vi "WindowLockMonitor.vi"() -> ()   [LabVIEW 2017]
uses:
  <vilib>/Platform/TimedLoop/XDataNode/timing_clust.ctl
  <vilib>/Platform/TimedLoop/XDataNode/nitl_modes.ctl
  <vilib>/Platform/TimedLoop/XDataNode/wakeup.ctl
  <vilib>/DAQmx/read.llb/DAQmx Read (Analog 1D DBL NChan 1Samp).vi
  <vilib>/DAQmx/create/channels.llb/DAQmx Create Channel (AI-Current-Basic).vi
  <vilib>/DAQmx/create/channels.llb/DAQmx Create Channel (AI-Voltage-Basic).vi
  <vilib>/DAQmx/miscellaneous.llb/DAQmx Fill In Error Info.vi
  <vilib>/platform/TimedLoop/XDataNode/XDataNode.xnode
  <vilib>/Platform/TimedLoop/XDataNode/XDNodeRunTimeDep.lvlib
panel:
  out "Distance":dbl format="%#_6f"
  out "Volte L2":dbl(graph)
  out "Volte L1":dbl(graph)
  out "Distance":dbl(graph)
  out "Force":dbl(graph)
  out "error out 2":errorcluster
  in  "stop":bool
  out "error out":errorcluster
  # "A."
  # "A."
  # "mm."
  # "V"
  # "V"
  # "WINDOW LOCK/UNLOCK"
  # "WINDOW LOCK/UNLOCK"
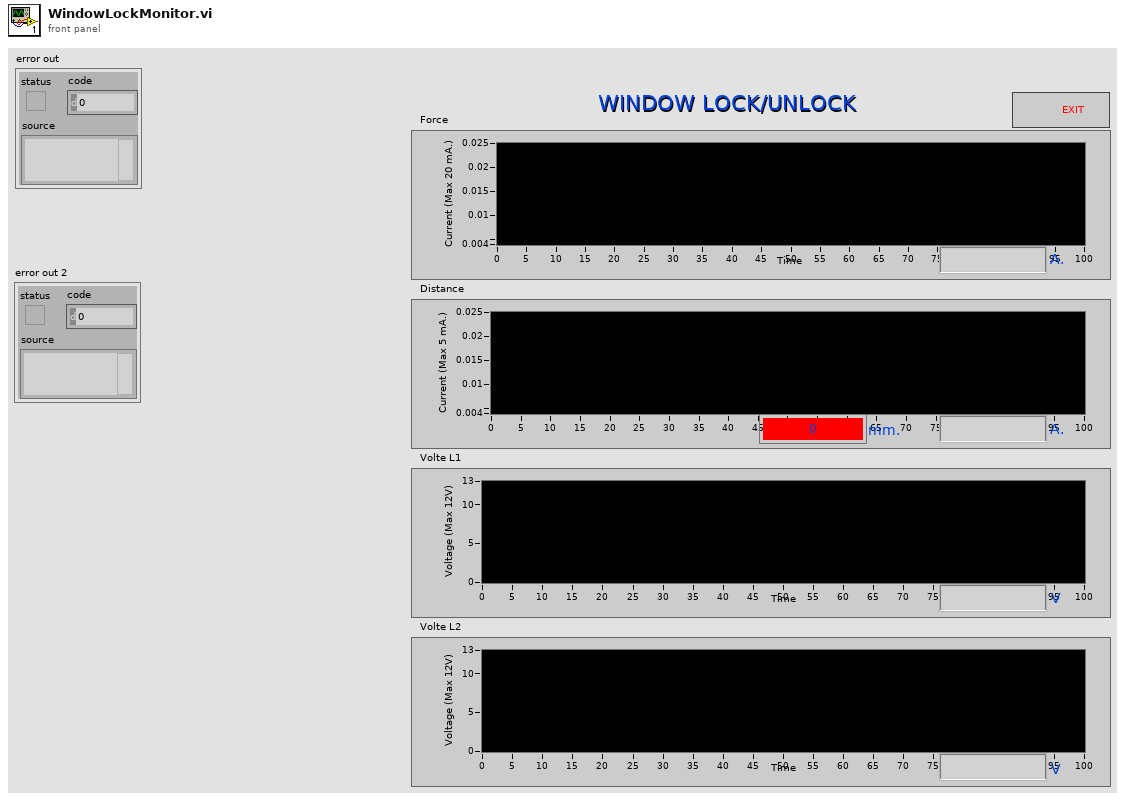
[diagram p1: front panel]
types:
  T1 = typedef "XDNodeRunTimeDep.lvlib/timing_clust.ctl" = cluster{"Expected End [f-1]":u64, "Actual End [f-1]":u64, "Finished Late? [f-1]":bool, "Expected End [i-1]":u64, "Actual End [i-1]":u64, "Finished Late? [i-1]":bool, "Expected Start [i]":u64, "Actual Start [i]":u64, "Expected Start [f]":u64, "Actual Start [f]":u64, "Source Name":string, "Structure Name":string, "Period":i64, "Deadline":i64, "Offset":i64, "Start":i64, "Priority":i32, "Timeout":i32, "Mode":T2, "Wakeup Reason":T3, "Error":errorcluster, "Source Type":string, "Secondary Source Type":string, "Global End Time":u64, "Global Start Time":u64, "Frame Duration":u64, "Iteration Duration":u64, "Assigned CPU":i32, "I/O Scan Engine Mode":u32}
  T2 = typedef "XDNodeRunTimeDep.lvlib/nitl_modes.ctl" = enum32{"No Change", "Process missed periods, maintain original phase", "Discard missed periods, maintain original phase", "Process missed periods, ignore original phase", "Discard missed periods, ignore original phase"}
  T3 = typedef "XDNodeRunTimeDep.lvlib/wakeup.ctl" = enum32{"Normal", "Aborted", "Asynchronous wakeup", "Timing source error", "Timed loop error", "Timeout"}
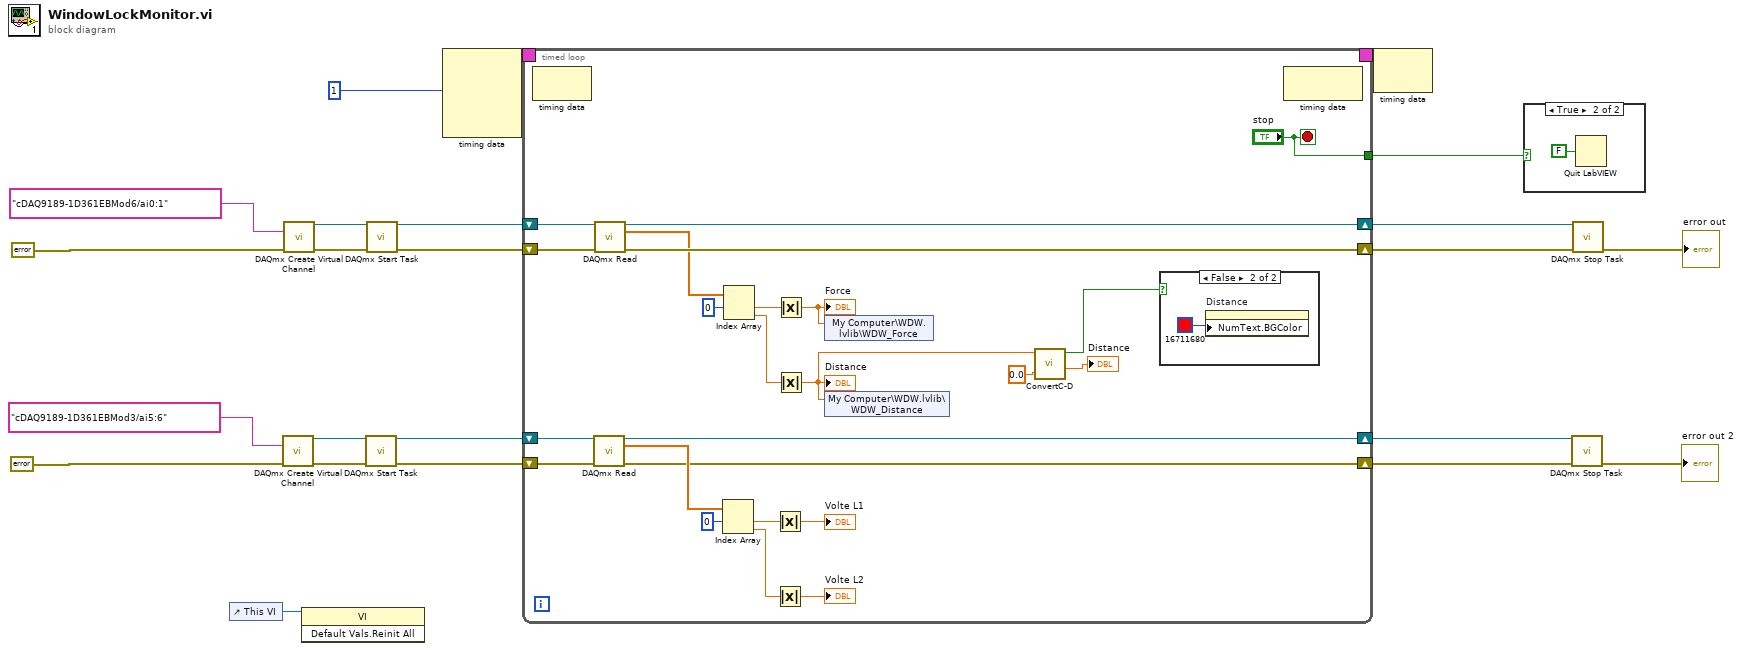
[diagram p0: block diagram]
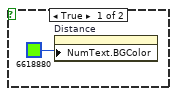
[diagram p3: hidden frame]
diagram:
  n1 = control-ref of="This VI"() -> (w11:refnum<vi>)
  n2 = call-poly <vilib>:"DAQmx Create Virtual Channel.vi"("physical channels"=tag "cDAQ9189-1D361EBMod3/ai5:6", "error in"=errorcluster {"status"=FALSE, "code"=0, "source"=""} ("error constant")) -> ("task out"=w6:refnum<k21>, "error out"=w7:errorcluster)  [unwired: 12 in]
  n3 = call-poly <vilib>:"DAQmx Create Virtual Channel.vi"("physical channels"=tag "cDAQ9189-1D361EBMod6/ai0:1", "error in"=errorcluster {"status"=FALSE, "code"=0, "source"=""} ("error constant")) -> ("task out"=w22:refnum<k21>, "error out"=w21:errorcluster)  [unwired: 12 in]
  n4 = invoke class="VI" method="Default Vals.Reinit All"(reference=w11) -> ()  [unwired: 2 in, 3 out]
  n5 = call <vilib>:"DAQmx Start Task.vi"("task/channels in"=w6, "error in"=w7) -> ("task out"=w4:refnum<k21>, "error out"=w3:errorcluster)  [unwired: 12 in]
  n6 = call <vilib>:"DAQmx Start Task.vi"("task/channels in"=w22, "error in"=w21) -> ("task out"=w20:refnum<k21>, "error out"=w19:errorcluster)  [unwired: 12 in]
  n7 = node-c288(i64 1 ("Period")) -> (w15:T1)  [unwired: 3 in]
  n8 = timed-loop {
    timing: w15 -> [_]
    timing-out: [_] -> w14
    shift-right: [w45] -> w17
    shift-left: w20 -> [w47]
    shift-right: [w44] -> w16
    shift-left: w19 -> [w46]
    tunnel: ["stop"] -> w10
    shift-right: [w32] -> w2
    shift-left: w4 -> [w34]
    shift-right: [w31] -> w1
    shift-left: w3 -> [w33]
    stop <- "stop" stop-if-true
    n9 = node-c288() -> ()  [unwired: 1 in, 1 out]
    n10 = call-poly <vilib>:"DAQmx Read.vi"("task/channels in"=w34, "error in"=w33) -> ("task out"=w32:refnum<k21>, "data"=w36:dbl[], "error out"=w31:errorcluster)  [unwired: 11 in]
    n11 = call-poly <vilib>:"DAQmx Read.vi"("task/channels in"=w47, "error in"=w46) -> ("task out"=w45:refnum<k21>, "data"=w42:dbl[], "error out"=w44:errorcluster)  [unwired: 11 in]
    n12 = Index Array(array=w36, index #1=0 ("index")) -> (element #1=w35:dbl, element #2=w38:dbl)  [unwired: 1 in]
    n13 = Index Array(array=w42, index #1=0 ("index")) -> (element #1=w43:dbl, element #2=w39:dbl)  [unwired: 1 in]
    n14 = Absolute Value(x=w35) -> (abs(x)=→"Volte L1":dbl)
    n15 = Absolute Value(x=w38) -> (abs(x)=→"Volte L2":dbl)
    n16 = Absolute Value(x=w43) -> (abs(x)=w28:dbl)
    "Force" <- w28
    n17 = Absolute Value(x=w39) -> (abs(x)=w27:dbl)
    "Distance" <- w27
    n18 = shared-variable "My Computer\\WDW.lvlib\\WDW_Force"(w28) -> ()  [unwired: 1 in, 1 out]
    n19 = shared-variable "My Computer\\WDW.lvlib\\WDW_Distance"(w27) -> ()  [unwired: 1 in, 1 out]
    n20 = call "ConvertC-D.vi"("Tolerance"=0.0, "Distance(mA.)"=w27) -> ("NormalDistance(mm.)"=→"Distance":dbl, "In Range?"=w24:bool)  [unwired: 6 in, 2 out]
    n21 = case shown="False" w24 {
      frame True {
        n22 = property on="Distance" class="DigNum (strict)"("NumText.BGColor"=u32 6618880) -> ()  [unwired: 2 in, 2 out]
      }
      frame False {
        n23 = property on="Distance" class="DigNum (strict)"("NumText.BGColor"=u32 16711680) -> ()  [unwired: 2 in, 2 out]
      }
    }
    n24 = node-c288() -> ()  [unwired: 1 in, 1 out]
  }
  n25 = node-c288(w14) -> ()  [unwired: 1 out]
  n26 = case shown="True" w10 {
    frame False {
    }
    frame True {
      n27 = Quit LabVIEW(quit? (T)=FALSE) -> ()
    }
  }
  n28 = call <vilib>:"DAQmx Stop Task.vi"("task/channels in"=w2, "error in"=w1) -> ("error out"=→"error out 2":errorcluster)  [unwired: 12 in, 1 out]
  n29 = call <vilib>:"DAQmx Stop Task.vi"("task/channels in"=w17, "error in"=w16) -> ("error out"=→"error out":errorcluster)  [unwired: 12 in, 1 out]
